vi "PCO_GetSensorDarkOffset.vi"(8 "error in (no error)":errorcluster {"code" format="%x"}, 11 "ph":u64) -> (0 "error out":errorcluster {"code" format="%x"}, 1 "wDarkOffset":u16, 2 "ErrorMessage":i32 format="%x", 3 "ph out":u64)   [LabVIEW 2020, in "SDK.lvlib" / "ImageSensor.lvlib"]
doc: "<b>Description:</b>\nGets the sensor dark offset.\n\n<b>Supported camera type:</b>\nAll\n\n<b>Descriptor dependency:</b>\nNone"
uses:
  ImageSensor.lvlib
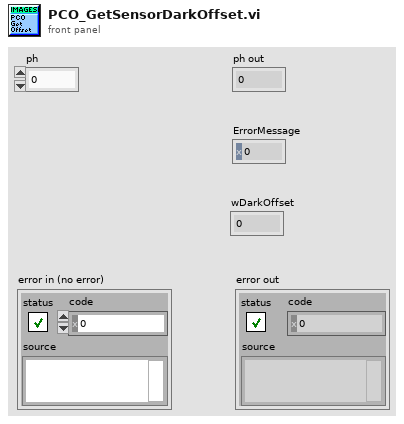
[diagram p1: front panel]
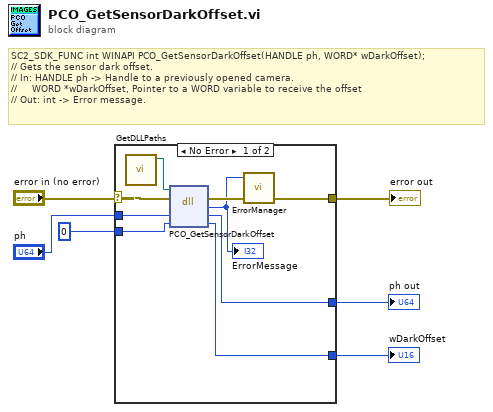
[diagram p0: block diagram]
diagram:
  # "SC2_SDK_FUNC int WINAPI PCO_GetSensorDarkOffset(HANDLE ph, WORD* wDarkOffset);\n// Gets the sensor dark offset.\n// In: HANDLE ph -> Handle to a previously opened camera.\n//     WORD *wDarkOffset, Pointer to a WORD variable to receive the offset\n// Out: int -> Error message."
  n1 = case shown="No Error" "error in (no error)" {
    selector: "error in (no error)" -> [w9 w18]
    tunnel: "ph" -> [w15 w17]
    tunnel: [w14 w17] -> w5
    tunnel: u16 0 ("wOffsetRegulation") -> [w13 w16]
    tunnel: [w12 w16] -> w3
    tunnel: [w10 w18] -> w2
    frame No Error {
      n2 = call "GetDLLPaths.vi"() -> ("SC2_Cam_Path"=w7:path)  [unwired: 9 in, 2 out]
      n3 = dll-call lib="?" fn="PCO_GetSensorDarkOffset"(path in=w7, error in=w9, "ph"=w15, "wDarkOffset"=w13) -> (error out=w11:errorcluster, "return type"=w8:i32, "ph"=w14:u64, "wDarkOffset"=w12:u16)  [unwired: 1 in, 1 out]
      "ErrorMessage" <- w8
      n4 = call "ErrorManager.vi"("error in (no error)"=w11, "error code"=w8) -> ("error out"=w10:errorcluster)  [unwired: 3 in]
    }
    frame Error {
    }
  }
  "ph out" <- w5
  "wDarkOffset" <- w3
  "error out" <- w2
